vi "Connect_EventRefOut_DBL.vi"(8 "Error In":errorcluster, 10 "Signal Signature":string, 11 "Sender In":refnum<class "LQObject.lvclass">) -> (0 "Error Out":errorcluster, 2 "DBL Signal":refnum<user-event>, 3 "Sender Out":refnum<class "LQObject.lvclass">)   [LabVIEW 2013, in "Template.lvlib" / "LQCoreEngine.lvclass"]
uses:
  LQCoreEngine.lvclass
  LQObject/LQObject.lvclass
  _Private/Signals and Slots/Connection Action.ctl
  LQIdentity/LQIdentity.lvclass/LQIdentity.ctl
  Template.lvlib
  LQIdentity/LQIdentity.lvclass
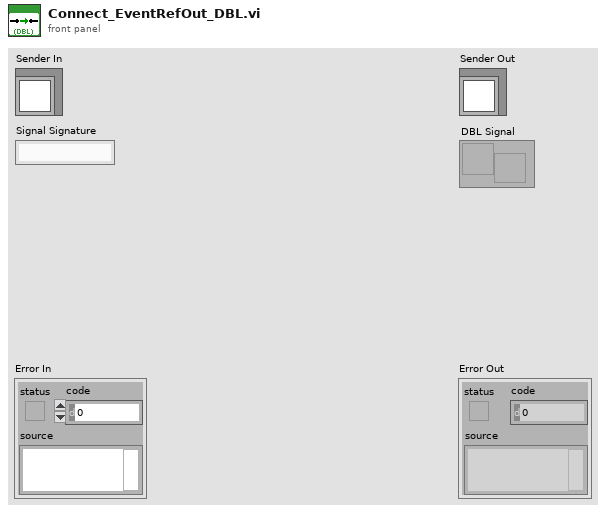
[diagram p1: front panel]
types:
  T1 = typedef "Template.lvlib/LQCoreEngine.lvclass/Connection Action.ctl" = enum16{"Init", "Add Connection", "Get Connections", "Clean Up"}
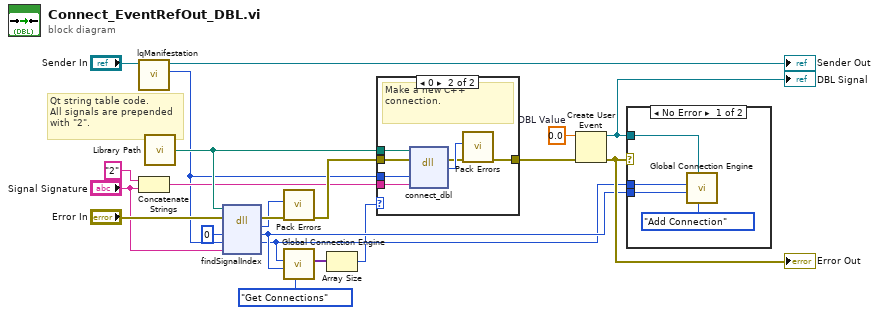
[diagram p0: block diagram]
diagram:
  w4 = 0.0  # DBL Value
  # "Qt string table code.\nAll signals are prepended\nwith \"2\"."
  n1 = call "lqManifestation.vi"("LQIdentity in"="Sender In") -> ("Manifestation"=w12:u64, "LQIdentity out"=→"Sender Out":refnum<class "LQObject.lvclass">)  [unwired: 9 in]
  n2 = Concatenate Strings("2" ("string"), "Signal Signature") -> (w14:string)
  n3 = call "Library Path.vi"() -> ("Library Path"=w18:path)
  n4 = dll-call lib="?" fn="findSignalIndex"(path in=w18, error in="Error In", "_retVal"=i64 0 ("retVal"), "_instance"=w12, "normalizedSignal"="Signal Signature") -> (error out=w10:errorcluster, "errorCode"=w9:i32, "_retVal"=w7:i64, "_instance"=w6:u64)  [unwired: 2 in, 1 out]
  n5 = call "Pack Errors.vi"("Error In"=w10, "Error Code"=w9) -> ("Error Out"=w20:errorcluster)  [unwired: 9 in]
  n6 = call "Global Connection Engine.vi"("Connection Action"=Connection_Action."Get Connections", "Signal Index"=w7, "QObject Refnum"=w6) -> ("Signal Channels"=w5:variant[])  [unwired: 8 in]
  n7 = Array Size(array=w5) -> (size(s)=w2:i32)
  n8 = case shown="0" w2 {
    tunnel: w14 -> [_ w29]
    tunnel: w18 -> [_ w28]
    tunnel: w12 -> [_ w27]
    tunnel: w20 -> [w22 w26]
    tunnel: [w22 w23] -> w3
    frame Default {
      # "Don't create a duplicate\nconnection."
    }
    frame 0 {
      # "Make a new C++\nconnection."
      n9 = dll-call lib="?" fn="connect_dbl"(path in=w28, error in=w26, "_instance"=w27, "encodedSignal"=w29) -> (error out=w24:errorcluster, "errorCode"=w25:i32)  [unwired: 3 in, 1 out]
      n10 = call "Pack Errors.vi"("Error In"=w24, "Error Code"=w25) -> ("Error Out"=w23:errorcluster)  [unwired: 9 in]
    }
  }
  n11 = Create User Event(user event datatype=w4, error in=w3) -> (user event=w1:refnum<user-event>, error out=w21:errorcluster)
  "Error Out" <- w21
  "DBL Signal" <- w1
  n12 = case shown="No Error" w21 {
    tunnel: w1 -> [w30 _]
    tunnel: w7 -> [w33 _]
    tunnel: w6 -> [w32 _]
    frame No Error {
      n13 = call "Global Connection Engine.vi"("Connection Action"=Connection_Action."Add Connection", "Signal Channel"=w30, "Signal Index"=w33, "QObject Refnum"=w32) -> ()  [unwired: 7 in, 1 out]
    }
    frame Error {
    }
  }
